vi "Configure Frequencies.vi"(3 "OSC Configuration In":T1(array[cluster])=[[{"Signal Type"=enum."Sine Wave", "DC"=0.0, "Amplitude"=0.001, "frequency"=2.0, "Phase"=0.0}, {"Signal Type"=enum."Sine Wave", "DC"=0.0, "Amplitude"=0.0, "frequency"=2.0, "Phase"=0.0}, {"Signal Type"=enum."Sine Wave", "DC"=0.0, "Amplitude"=0.0, "frequency"=20.0, "Phase"=0.0}], [{"Signal Type"=enum."Sine Wave", "DC"=0.0, "Amplitude"=0.0, "frequency"=2.0, "Phase"=0.0}, {"Signal Type"=enum."Sine Wave", "DC"=0.0, "Amplitude"=0.0, "frequency"=2.0, "Phase"=0.0}, {"Signal Type"=enum."Sine Wave", "DC"=0.0, "Amplitude"=0.0, "frequency"=20.0, "Phase"=0.0}]] {"frequency" step=0.001 format="%.3p"; "Amplitude" format="%0.2p"; "DC" min=-0.99 max=0.99 format="%.2p"}) -> (0 "Frequency Out":dbl, 1 "OSC Configuation Out":T1(array[cluster]))   [LabVIEW 2011, in "Lock-In Variable Channels_2.lvclass"]
uses:
  Lock-In Variable Channels_2.lvclass
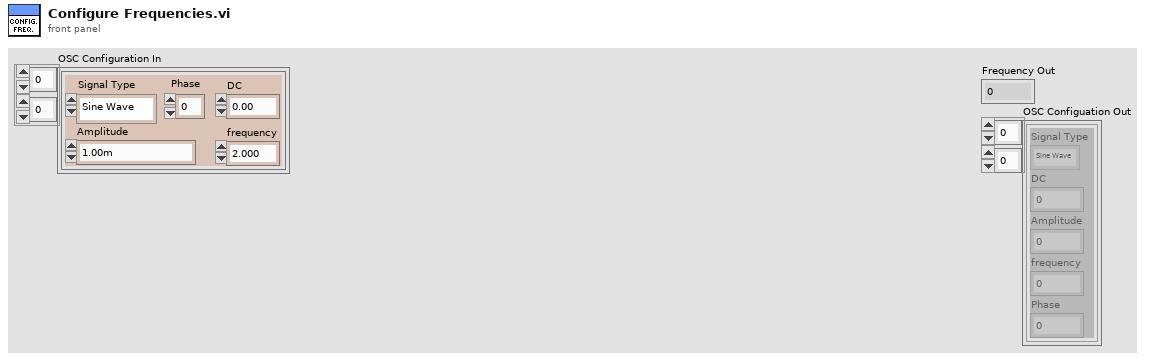
[diagram p1: front panel]
types:
  T1 = cluster{"Signal Type":enum16{"Sine Wave", "Triangle Wave", "Square Wave", "Sawtooth Wave"}, "DC":dbl, "Amplitude":dbl, "frequency":dbl, "Phase":dbl}[][]
  T2 = cluster{"Signal Type":enum16{"Sine Wave", "Triangle Wave", "Square Wave", "Sawtooth Wave"}, "DC":dbl, "Amplitude":dbl, "frequency":dbl, "Phase":dbl}
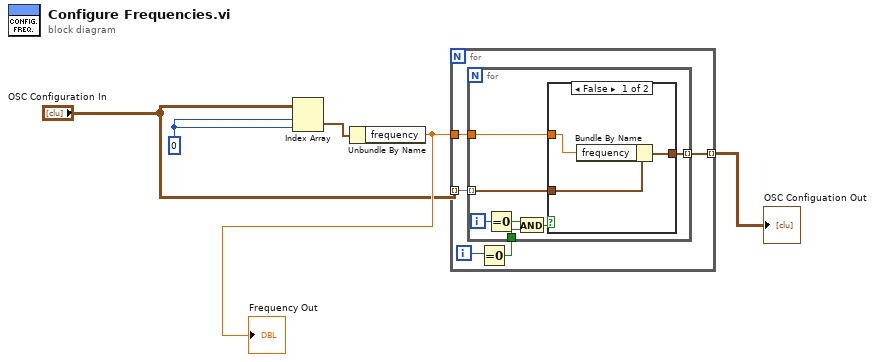
[diagram p0: block diagram]
diagram:
  w5 = 0 ("disabled index (col)")
  n1 = Index Array(array="OSC Configuration In", index (row)=w5, index (col)=w5) -> (element=w2:T2)
  n2 = Unbundle By Name(w2) -> ("frequency"=w3:dbl)
  "Frequency Out" <- w3
  n3 = for {
    tunnel: "OSC Configuration In" -> [w10] mode=indexing
    tunnel: w3 -> [w9]
    tunnel: [w8] -> w4 mode=indexing
    i -> [w7]
    n4 = Equal To 0?(x=w7) -> (x = 0?=w6:bool)
    n5 = for {
      tunnel: w10 -> [w17] mode=indexing
      tunnel: w9 -> [w16]
      tunnel: [w15] -> w8 mode=indexing
      tunnel: w6 -> [w12]
      i -> [w14]
      n6 = Equal To 0?(x=w14) -> (x = 0?=w13:bool)
      n7 = And(x=w13, y=w12) -> (x .and. y?=w11:bool)
      n8 = case shown="False" w11 {
        tunnel: w17 -> [w20 w21]
        tunnel: w16 -> [w19 _]
        tunnel: [w18 w21] -> w15
        frame False {
          n9 = Bundle By Name(cluster=w20, "frequency"=w19) -> (w18:T2)
        }
        frame True {
        }
      }
    }
  }
  "OSC Configuation Out" <- w4
